vi "LEP_RV_MemoryMap_GetMemConfig.vi"(8 "error in (no error)":errorcluster, 11 "Source File":path) -> (0 "error out":errorcluster, 1 "Mem Config String":string, 2 "Code Section":string, 3 "Data Section":string)   [LabVIEW 2011]
doc: "Query memory mapper database for the memory section the passed VI should be placed in."
uses:
  LEP_RV_MemoryMap_Sections.ctl
panel:
  out "Data Mem":i32
  out "Code Mem":i32
  in  "vi file names":path[](array[path])
  in  "c file names":string[](array[string])
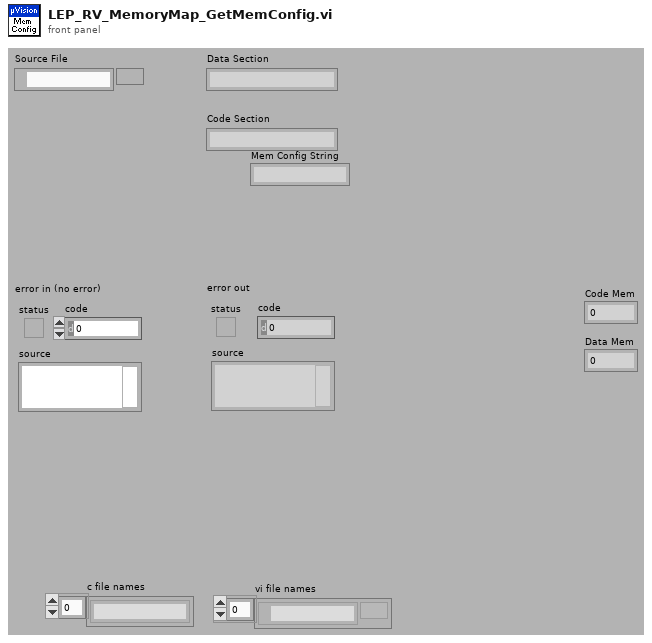
[diagram p1: front panel]
types:
  T1 = typedef "EMB_Utility_MemMap_VI_Config.ctl" = cluster{"filename":string, "Code Section":i32, "Code Section List":i32[], "Const Section":i32, "Const Section List":i32[], "VI Type":T2}
  T2 = typedef "EMB_Utility_MemMap_VI_Type.ctl" = enum32{"invalid VI type", "Standard VI", "Control VI", "Global VI", "Polymorphic VI", "Configuration VI", "SubSystem"}
  T3 = typedef "LEP_RV_MemoryMap_Sections.ctl" = enum16{"ROM1 (0)", "ROM2 (1)", "ROM3 (2)", "IROM1 (3)", "IROM2 (4)", "RAM1 (5)", "RAM2 (6)", "RAM3 (7)", "IRAM1 (8)", "IRAM2 (9)"}
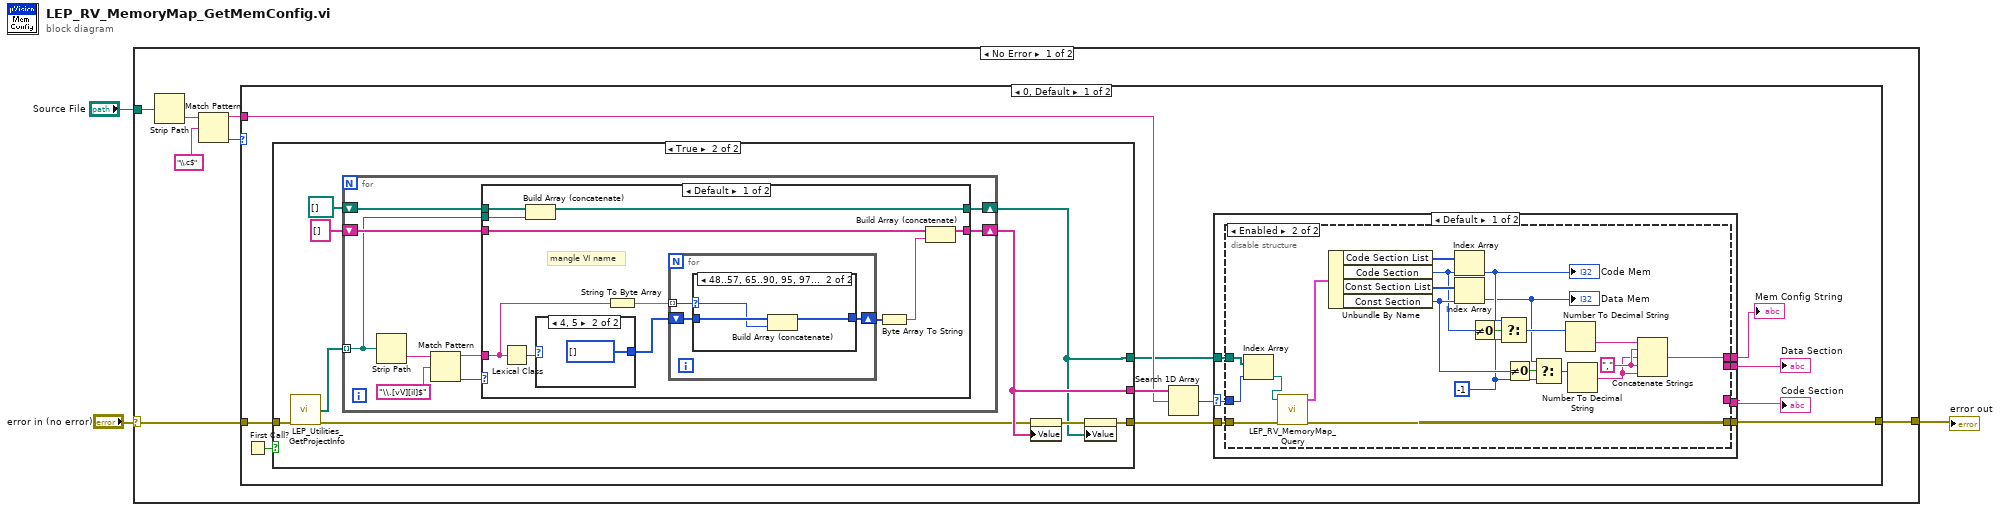
[diagram p0: block diagram]
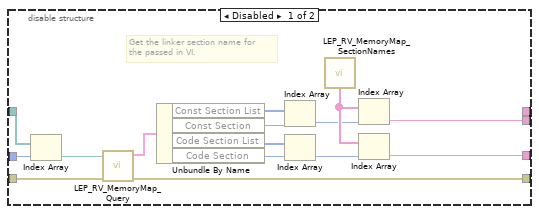
[diagram p2: hidden frame]
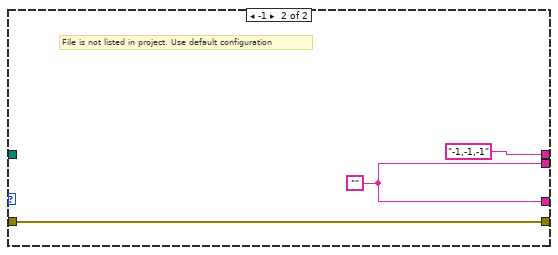
[diagram p3: hidden frame]
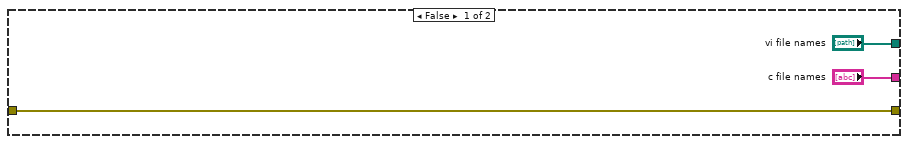
[diagram p4: hidden frame]
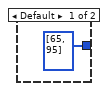
[diagram p5: hidden frame]
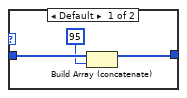
[diagram p6: hidden frame]
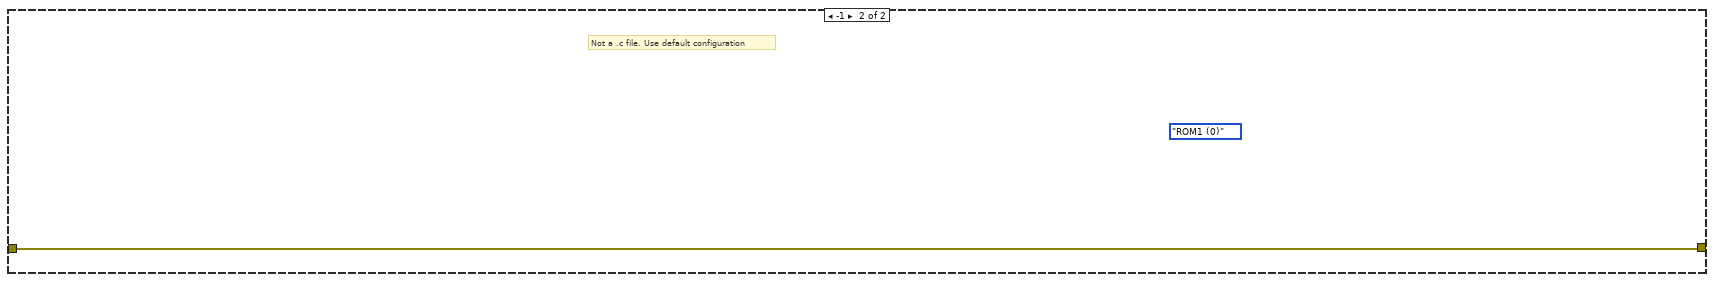
[diagram p8: hidden frame]
diagram:
  n1 = case shown="No Error" "error in (no error)" {
    selector: "error in (no error)" -> [w9 w114]
    tunnel: "Source File" -> [w10 _]
    tunnel: [w8 w114] -> w1
    frame No Error {
      n2 = Strip Path(path=w10) -> (name=w7:string)  [unwired: 1 out]
      n3 = Match Pattern(string=w7, regular expression="\\.c$") -> (before substring=w4:string, offset past match=w5:i32)  [unwired: 3 out]
      n4 = case shown="0, Default" w5 {
        tunnel: w4 -> [w15 _]
        tunnel: w9 -> [w21 w113]
        tunnel: [w16 w113] -> w8
        frame 0, Default {
          n5 = First Call?() -> (First Call?: T/F=w20:bool)
          n6 = case shown="True" w20 {
            tunnel: w21 -> [w69 w79]
            tunnel: [w69 w74] -> w17
            tunnel: ["c file names" w77] -> w19
            tunnel: ["vi file names" w71] -> w14
            frame False {
            }
            frame True {
              n7 = call <vilib>:"LEP_Utilities_GetProjectInfo.vi"("error in"=w79) -> ("SourceFiles"=w78:path[], "error out"=w75:errorcluster)  [unwired: 13 out]
              n8 = for {
                tunnel: w78 -> [w81] mode=indexing
                shift-right: [w84] -> w77
                shift-left: string[] [] -> [w85]
                shift-right: [w82] -> w71
                shift-left: path[] [] -> [w83]
                n9 = Strip Path(path=w81) -> (name=w80:string)  [unwired: 1 out]
                n10 = Match Pattern(string=w80, regular expression="\\.[vV][iI]$") -> (before substring=w86:string, offset past match=w87:i32)  [unwired: 3 out]
                n11 = case shown="Default" w87 {
                  tunnel: w86 -> [w90 _]
                  tunnel: w85 -> [w95 w112]
                  tunnel: [w94 w112] -> w84
                  tunnel: [w91 w111] -> w82
                  tunnel: w83 -> [w92 w111]
                  tunnel: w81 -> [w89 _]
                  frame Default {
                    # "mangle VI name"
                    n12 = Lexical Class(1:w90) -> (0:w97:i16)
                    n13 = Build Array (concatenate)(w92, w89) -> (w91:path[])
                    n14 = case shown="4, 5" w97 {
                      tunnel: [u8[] [65, 95] ("unsigned byte array") u8[] [] ("unsigned byte array")] -> w96
                      frame Default {
                      }
                      frame 4, 5 {
                      }
                    }
                    n15 = String To Byte Array(string=w90) -> (unsigned byte array=w99:u8[])
                    n16 = for {
                      tunnel: w99 -> [w103] mode=indexing
                      shift-right: [w102] -> w98
                      shift-left: w96 -> [w104]
                      n17 = case shown="48..57, 65..90, 95, 97..122" w103 {
                        selector: w103 -> [_ w109]
                        tunnel: w104 -> [w107 w110]
                        tunnel: [w106 w108] -> w102
                        frame Default {
                          n18 = Build Array (concatenate)(w107, u8 95) -> (w106:u8[])
                        }
                        frame 48..57, 65..90, 95, 97..122 {
                          n19 = Build Array (concatenate)(w110, w109) -> (w108:u8[])
                        }
                      }
                    }
                    n20 = Byte Array To String(unsigned byte array=w98) -> (string=w93:string)
                    n21 = Build Array (concatenate)(w95, w93) -> (w94:string[])
                  }
                  frame -1 {
                  }
                }
              }
              n22 = property on="c file names" class="Arr (strict)"(error in=w75, "Value"=w77) -> (error out=w72:errorcluster)  [unwired: 1 in, 1 out]
              n23 = property on="vi file names" class="Arr (strict)"(error in=w72, "Value"=w71) -> (error out=w74:errorcluster)  [unwired: 1 in, 1 out]
            }
          }
          n24 = Search 1D Array(1D array=w19, element=w15) -> (index of element=w18:i32)  [unwired: 1 out]
          n25 = case shown="Default" w18 {
            selector: w18 -> [w26 _]
            tunnel: w17 -> [w28 w67]
            tunnel: [w27 w67] -> w16
            tunnel: w14 -> [w25 _]
            tunnel: [w24 w66] -> w13
            tunnel: [w23 w66] -> w12
            tunnel: [w22 "-1,-1,-1"] -> w11
            frame Default {
              n26 = disable-structure shown="Enabled" {
                disable-tunnel: w28 -> [w42 w58]
                disable-tunnel: [w41 w54] -> w27
                disable-tunnel: w26 -> [w40 w56]
                disable-tunnel: w25 -> [w39 w57]
                disable-tunnel: [w37 _] -> w24
                disable-tunnel: [w36 _] -> w23
                disable-tunnel: [_ w53] -> w22
                frame Disabled {
                  # "Get the linker section name for\nthe passed in VI."
                  n27 = Index Array(array=w39, index=w40) -> (element=w29:path)
                  n28 = call "LEP_RV_MemoryMap_Query.vi"("error in (no error)"=w42, "Source File"=w29) -> ("error out"=w41:errorcluster, "VI Config"=w43:T1)  [unwired: 8 in]
                  n29 = Unbundle By Name(w43) -> ("Const Section List"=w35:i32[], "Const Section"=w34:i32, "Code Section List"=w32:i32[], "Code Section"=w31:i32)
                  n30 = Index Array(array=w35, index=w34) -> (element=w33:i32)
                  n31 = Index Array(array=w32, index=w31) -> (element=w30:i32)
                  n32 = call "LEP_RV_MemoryMap_SectionNames.vi"() -> ("Linker Names"=w38:string[])  [unwired: 2 in, 1 out]
                  n33 = Index Array(array=w38, index=w33) -> (element=w37:string)
                  n34 = Index Array(array=w38, index=w30) -> (element=w36:string)
                }
                frame Enabled {
                  w44 = -1 ("f")
                  w61 = "," ("string")
                  n35 = Index Array(array=w57, index=w56) -> (element=w55:path)
                  n36 = call "LEP_RV_MemoryMap_Query.vi"("error in (no error)"=w58, "Source File"=w55) -> ("error out"=w54:errorcluster, "VI Config"=w64:T1)  [unwired: 8 out]
                  n37 = Unbundle By Name(w64) -> ("Code Section List"=w63:i32[], "Code Section"=w45:i32, "Const Section List"=w62:i32[], "Const Section"=w46:i32)
                  n38 = Index Array(array=w63, index=w45) -> (element=w52:i32)
                  "Code Mem" <- w52
                  n39 = Index Array(array=w62, index=w46) -> (element=w48:i32)
                  "Data Mem" <- w48
                  n40 = Not Equal To 0?(x=w45) -> (x != 0?=w51:bool)
                  n41 = Select(t=w52, s=w51, f=w44) -> (s? t:f=w49:i32)
                  n42 = Not Equal To 0?(x=w46) -> (x != 0?=w50:bool)
                  n43 = Select(t=w48, s=w50, f=w44) -> (s? t:f=w47:i32)
                  n44 = Number To Decimal String(number=w49) -> (decimal integer string=w60:string)  [unwired: 1 out]
                  n45 = Number To Decimal String(number=w47) -> (decimal integer string=w59:string)  [unwired: 1 out]
                  n46 = Concatenate Strings(w60, w61, w59, w61, w59) -> (w53:string)
                }
              }
            }
            frame -1 {
              w66 = ""
              # "File is not listed in project. Use default configuration"
            }
          }
          "Data Section" <- w13
          "Code Section" <- w12
          "Mem Config String" <- w11
        }
        frame -1 {
          (unwired) LEP_RV_MemoryMap_Sections."ROM1 (0)" ("Section Type")
          # "Not a .c file. Use default configuration"
        }
      }
    }
    frame Error {
    }
  }
  "error out" <- w1
